vi "BuildErrorSource.vi"(8 "error in":errorcluster, 10 "status code":i32=1, 11 "extended error info":string) -> (0 "error out":errorcluster)   [LabVIEW 2015]
doc: "This subVI reads in an error description and creates a custom error code for that description between 5000 and 9000. The result should be fairly unique."
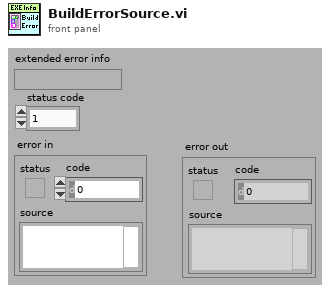
[diagram p1: front panel]
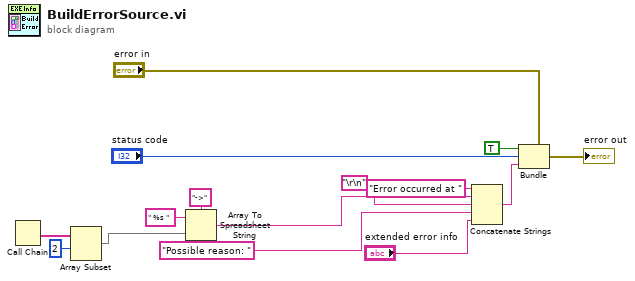
[diagram p0: block diagram]
diagram:
  n1 = Call Chain() -> (call chain=w4:string[])
  n2 = Array Subset(array=w4, index=2) -> (w2:string[])  [unwired: 1 in]
  n3 = Array To Spreadsheet String(delimiter (Tab)="->", array=w2, 3:" %s " ("format string")) -> (spreadsheet string=w7:string)
  n4 = Concatenate Strings("Error occurred at " ("string"), w7, "\r\n", "Possible reason: " ("string"), "extended error info") -> (w14:string)
  n5 = Bundle(cluster="error in", "status"=TRUE, "code"="status code", "source"=w14) -> (→"error out":errorcluster)
